vi "Case Ramp chart prop.vi"() -> ()   [LabVIEW 2012]
panel:
  in  "Y Scale.Grid Colors:Major Color":u32
  in  "X Scrollbar Visible":bool
  in  "Plot Area:Colors:BG Color":u32
  in  "Plot Area:Size:Height":u32
  in  "Frame Color":u32
  in  "X Scale.Grid Colors:Major Color":u32
  in  "X Scale.Scale Fit":u8
  in  "X Scale.Style":u8
  in  "X Scale.Range:Minor Increment":dbl
  in  "X Scale.Offset and Multiplier:Offset":dbl
  in  "X Scale.Visible":bool
  in  "X Scale.Range:Minimum":dbl
  out "time stamp":timestamp
  in  "Update Mode":u8
  out "XY Graph":cluster{"Y":dbl[], "Y":dbl[]}[](graph)
  out "Elapsed Time (s)":dbl
  out "Waveform Chart":cluster{"Elapsed Time (s)":dbl, "Result":dbl}(graph)
  in  "stop":bool
  out "Tank":dbl(slide) scale=0.0..10.0
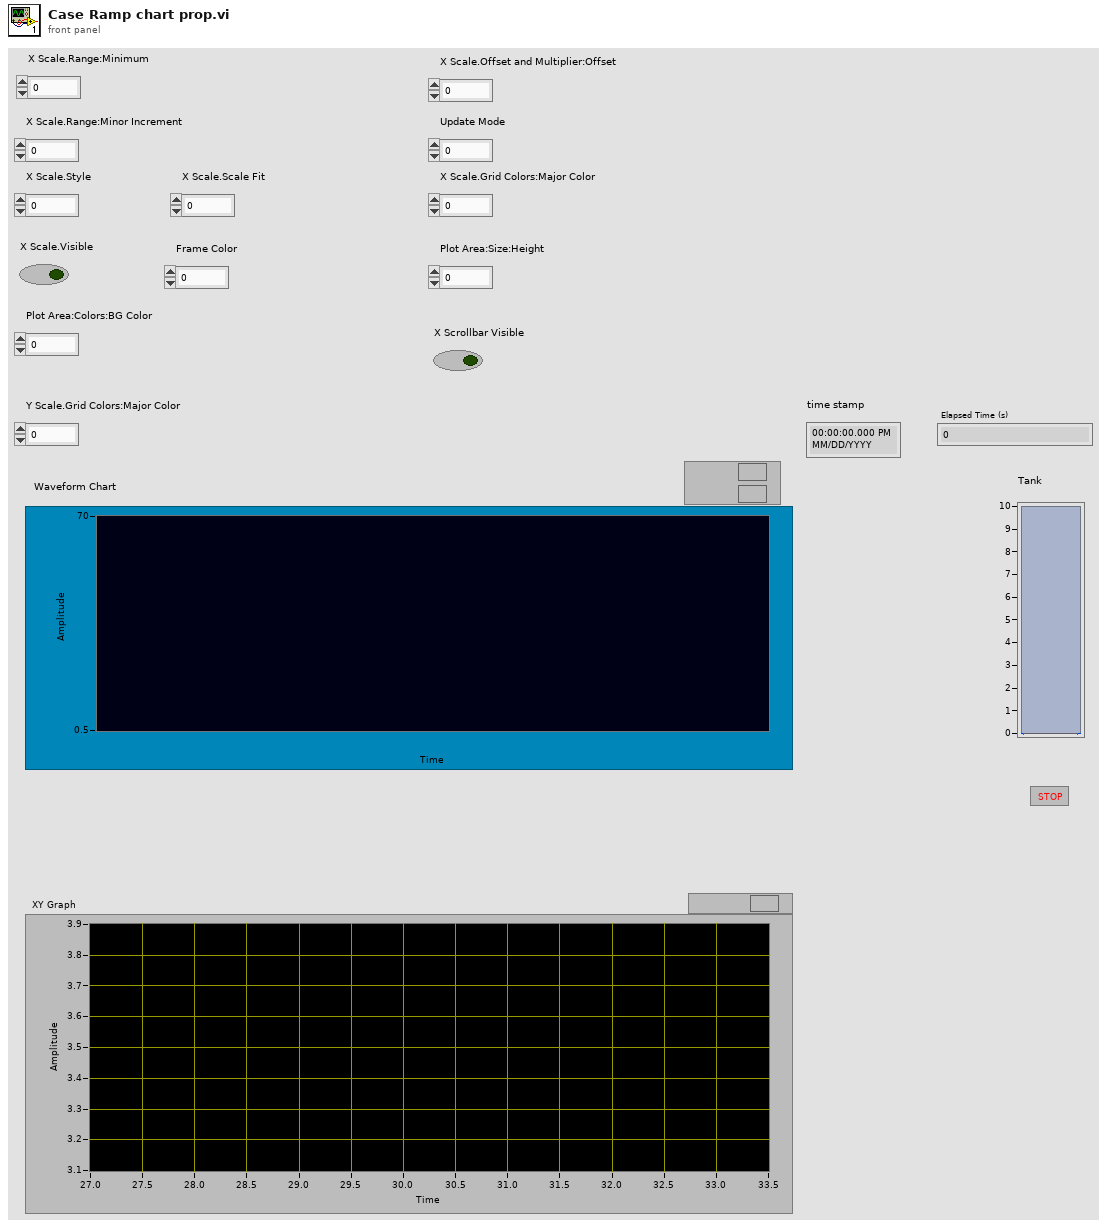
[diagram p1: front panel]
types:
  T1 = cluster{"second":i32, "minute":i32, "hour":i32, "day of month":i32, "month":i32, "year":i32, "day of week":i32, "day of year":i32, "is DST":i32}
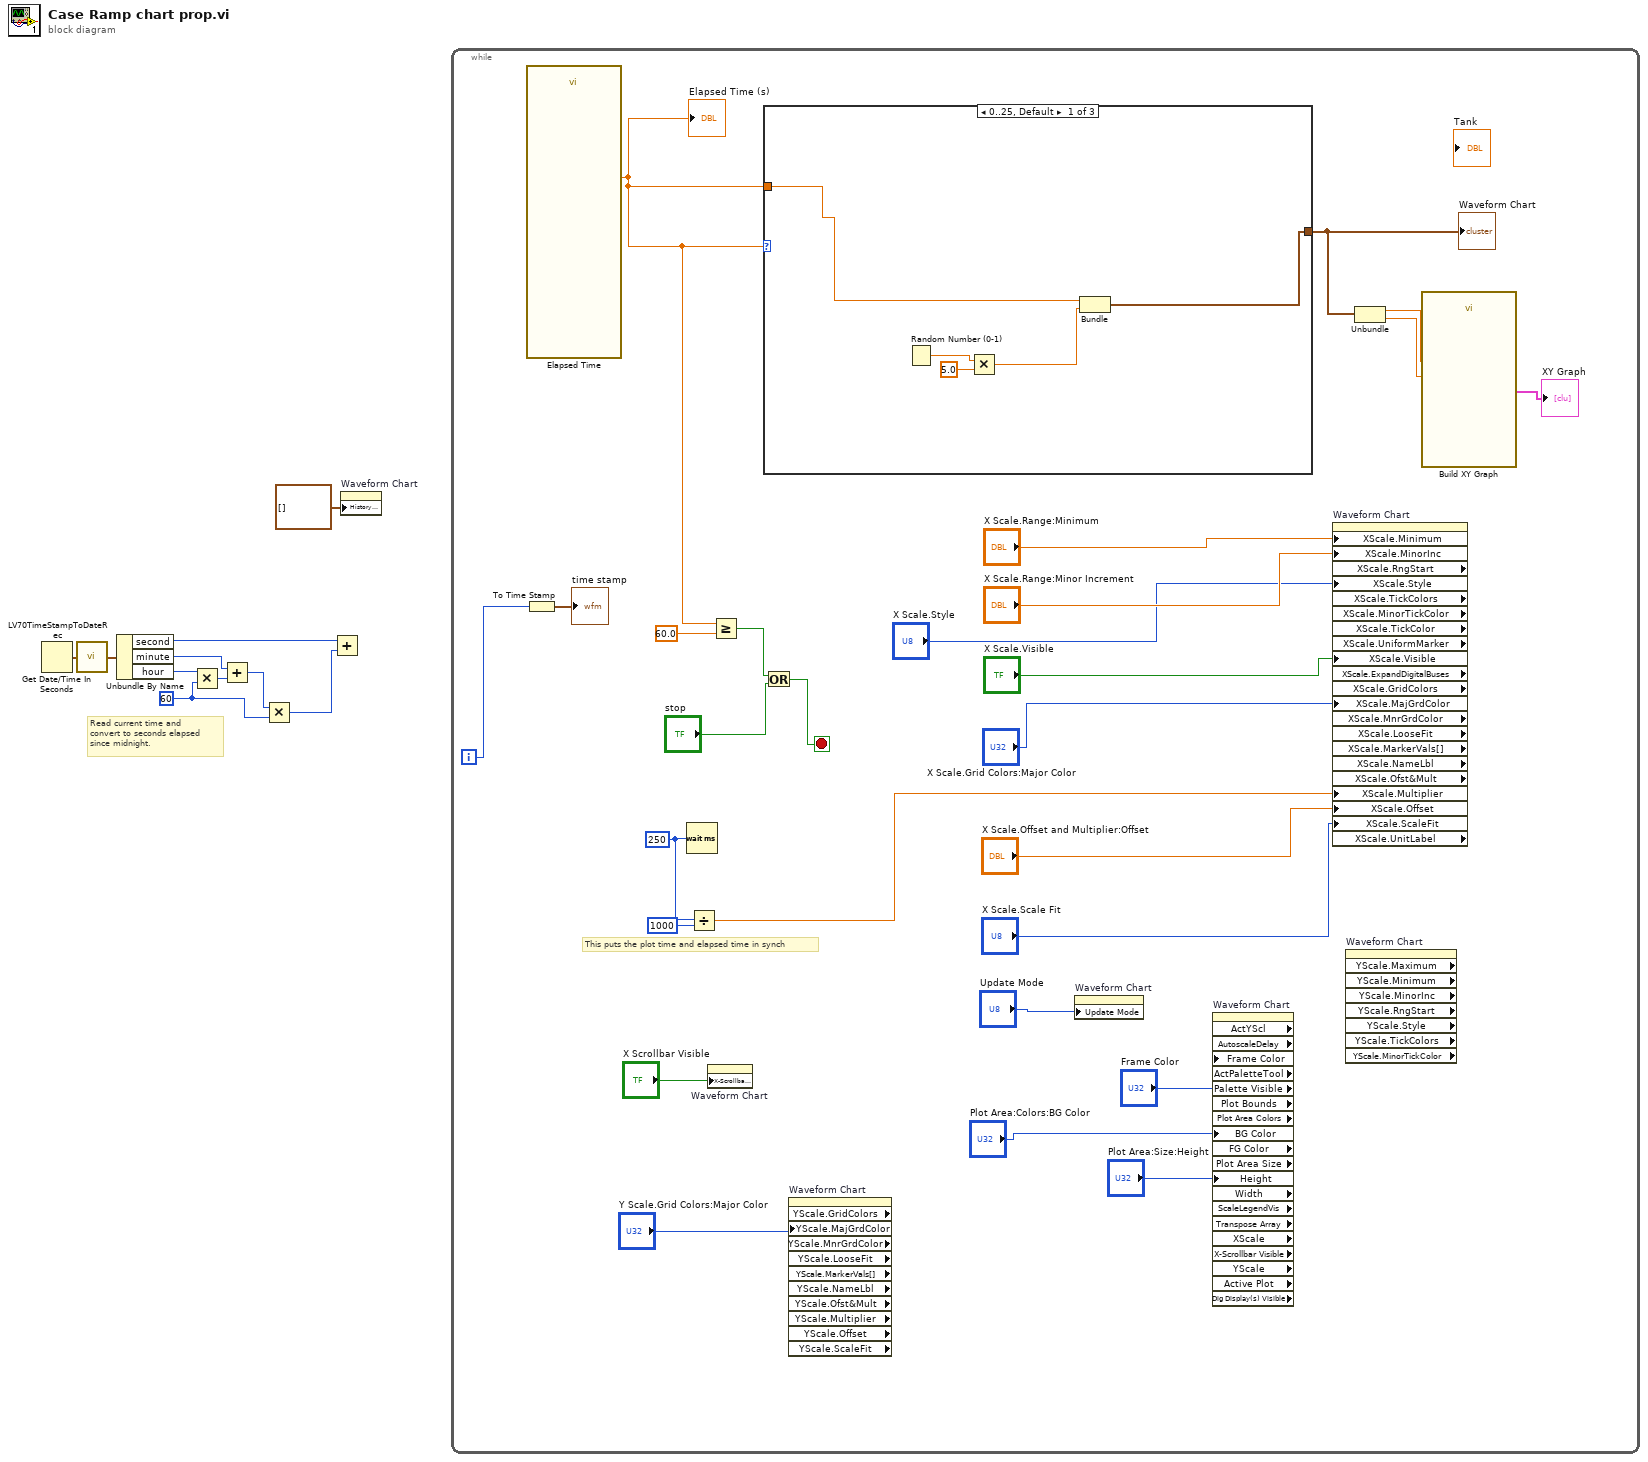
[diagram p0: block diagram]
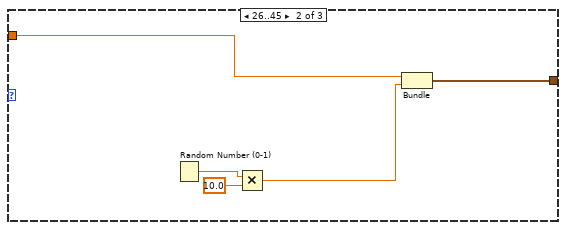
[diagram p2: hidden frame]
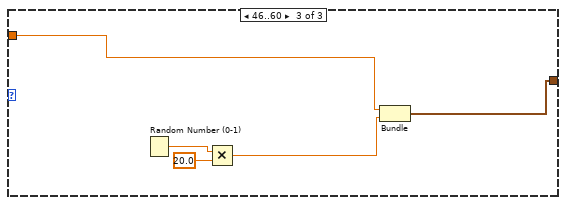
[diagram p3: hidden frame]
diagram:
  w2 = 60
  # "Read current time and\nconvert to seconds elapsed\nsince midnight."
  n1 = Get Date/Time In Seconds() -> (seconds since 1Jan1904=w1:timestamp)
  n2 = call <vilib>:"LV70TimeStampToDateRec.vi"("time stamp"=w1) -> ("date time rec"=w9:T1)
  n3 = Unbundle By Name(w9) -> ("second"=w3:i32, "minute"=w6:i32, "hour"=w8:i32)
  n4 = Multiply(x=w8, y=w2) -> (x*y=w7:i32)
  n5 = Add(x=w6, y=w7) -> (x+y=w5:i32)
  n6 = Multiply(x=w5, y=w2) -> (x*y=w4:i32)
  n7 = Add(x=w3, y=w4) -> ()  [unwired: 1 out]
  n8 = property on="Waveform Chart" class="WFChart (strict)"("History Data"=cluster{"Elapsed Time (s)":dbl, "Result":dbl}[] []) -> ()  [unwired: 2 in, 2 out]
  n9 = while {
    i -> [w27]
    stop <- w33 stop-if-true
    w22 = u32 250 ("milliseconds to wait")
    # "This puts the plot time and elapsed time in synch"
    n10 = call "Elapsed Time"() -> ("Elapsed Time (s)"=w36:dbl)  [unwired: 12 in, 7 out]
    "Elapsed Time (s)" <- w36
    n11 = To Time Stamp(1:w27) -> (0:→"time stamp":timestamp)
    n12 = Wait (ms)(milliseconds to wait=w22) -> ()  [unwired: 1 out]
    n13 = Divide(x=w22, y=u32 1000) -> (x/y=w20:dbl)
    n14 = property on="Waveform Chart" class="WFChart (strict)"("X-Scrollbar Visible"="X Scrollbar Visible") -> ()  [unwired: 2 in, 2 out]
    n15 = Greater Or Equal?(x=w36, y=60.0) -> (x >= y?=w34:bool)
    n16 = case shown="0..25, Default" w36 {
      tunnel: w36 -> [w42 w46 w52]
      tunnel: [w41 w47 w51] -> w31
      frame 0..25, Default {
        n17 = Random Number (0-1)() -> (number: 0 to 1=w40:dbl)
        n18 = Multiply(x=w40, y=5.0) -> (x*y=w38:dbl)
        n19 = Bundle("Elapsed Time (s)"=w42, w38) -> (w41:cluster{"Elapsed Time (s)":dbl, dbl})  [unwired: 1 in]
      }
      frame 26..45 {
        n20 = Random Number (0-1)() -> (number: 0 to 1=w45:dbl)
        n21 = Multiply(x=w45, y=10.0) -> (x*y=w43:dbl)
        n22 = Bundle("Elapsed Time (s)"=w46, w43) -> (w47:cluster{"Elapsed Time (s)":dbl, dbl})  [unwired: 1 in]
      }
      frame 46..60 {
        n23 = Random Number (0-1)() -> (number: 0 to 1=w50:dbl)
        n24 = Multiply(x=w50, y=20.0) -> (x*y=w48:dbl)
        n25 = Bundle("Elapsed Time (s)"=w52, w48) -> (w51:cluster{"Elapsed Time (s)":dbl, dbl})  [unwired: 1 in]
      }
    }
    "Waveform Chart" <- w31
    n26 = Or(x=w34, y="stop") -> (x .or. y?=w33:bool)
    n27 = property on="Waveform Chart" class="WFChart (strict)" props=["YScale", "GridColors", "YScale", "MajGrdColor", "YScale", "MnrGrdColor", "YScale", "LooseFit", "YScale", "MarkerVals[]", "YScale", "NameLbl", "YScale", "Ofst&Mult", "YScale", "Multiplier", "YScale", "Offset", "YScale", "ScaleFit"]("YScale.MajGrdColor"="Y Scale.Grid Colors:Major Color") -> ()  [unwired: 2 in, 11 out]
    n28 = property on="Waveform Chart" class="WFChart (strict)"("Update Mode"="Update Mode") -> ()  [unwired: 2 in, 2 out]
    n29 = property on="Waveform Chart" class="WFChart (strict)" props=["ActYScl", "AutoscaleDelay", "Frame Color", "ActPaletteTool", "Palette Visible", "Plot Bounds", "Plot Area Colors", "BG Color", "FG Color", "Plot Area Size", "Height", "Width", "ScaleLegendVis", "Transpose Array", "XScale", "X-Scrollbar Visible", "YScale", "Active Plot", "Dig Display(s) Visible"]("Frame Color"="Frame Color", "BG Color"="Plot Area:Colors:BG Color", "Height"="Plot Area:Size:Height") -> ()  [unwired: 2 in, 18 out]
    n30 = property on="Waveform Chart" class="WFChart (strict)" props=["XScale", "Minimum", "XScale", "MinorInc", "XScale", "RngStart", "XScale", "Style", "XScale", "TickColors", "XScale", "MinorTickColor", "XScale", "TickColor", "XScale", "UniformMarker", "XScale", "Visible", "XScale", "ExpandDigitalBuses", "XScale", "GridColors", "XScale", "MajGrdColor", "XScale", "MnrGrdColor", "XScale", "LooseFit", "XScale", "MarkerVals[]", "XScale", "NameLbl", "XScale", "Ofst&Mult", "XScale", "Multiplier", "XScale", "Offset", "XScale", "ScaleFit", "XScale", "UnitLabel"]("XScale.Minimum"="X Scale.Range:Minimum", "XScale.MinorInc"="X Scale.Range:Minor Increment", "XScale.Style"="X Scale.Style", "XScale.Visible"="X Scale.Visible", "XScale.MajGrdColor"="X Scale.Grid Colors:Major Color", "XScale.Multiplier"=w20, "XScale.Offset"="X Scale.Offset and Multiplier:Offset", "XScale.ScaleFit"="X Scale.Scale Fit") -> ()  [unwired: 2 in, 15 out]
    n31 = property on="Waveform Chart" class="WFChart (strict)" props=["YScale", "Maximum", "YScale", "Minimum", "YScale", "MinorInc", "YScale", "RngStart", "YScale", "Style", "YScale", "TickColors", "YScale", "MinorTickColor"]() -> ()  [unwired: 2 in, 9 out]
    n32 = Unbundle(w31) -> ("Elapsed Time (s)"=w30:dbl, w29:dbl)
    n33 = call "Build XY Graph"("Y Input"=w29, "X Input"=w30) -> ("XY Graph"=→"XY Graph":cluster{"Y":dbl[], "Y":dbl[]}[])  [unwired: 3 in, 6 out]
  }
